vi "TMT04014Circuit.vi"(11 "power_heater?":bool) -> (3 "heater_output":i16)   [LabVIEW 2020]
doc: "Converts a digital output into the heater power output."
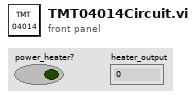
[diagram p1: front panel]
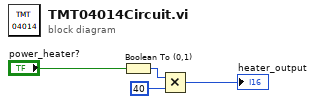
[diagram p0: block diagram]
diagram:
  n1 = Boolean To (0,1)(Boolean="power_heater?") -> (0, 1=w1:i16)
  n2 = Multiply(x=w1, y=i16 40) -> (x*y=→"heater_output":i16)
